vi "RangeCheck.vi"(8 "error in (no error)":errorcluster caption="エラー入力（エラーなし）", 10 "数値範囲チェック":T1={"デフォルト"=2.0, "最大値"=1.0, "最小値"=0.0}, 11 "数値文字列":string="0") -> (0 "error out":errorcluster caption="エラー出力", 2 "強制(x)":dbl, 3 "範囲内?(有効:TRUE,無効:FALSE)":bool)   [LabVIEW 2015]
uses:
  RangeCheck.ctl
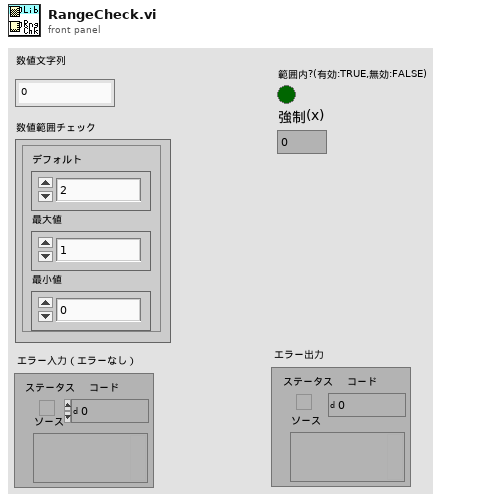
[diagram p1: front panel]
types:
  T1 = typedef "RangeCheck.ctl" = cluster{"デフォルト":dbl, "最大値":dbl, "最小値":dbl}
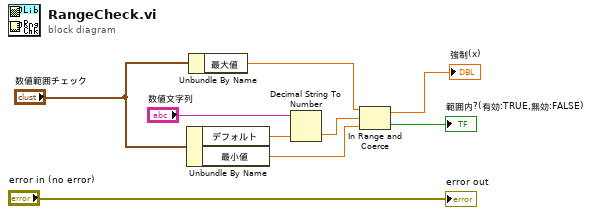
[diagram p0: block diagram]
diagram:
  n1 = Unbundle By Name("数値範囲チェック") -> ("デフォルト"=w9:dbl, "最小値"=w7:dbl)
  n2 = Unbundle By Name("数値範囲チェック") -> ("最大値"=w8:dbl)
  n3 = Decimal String To Number(string="数値文字列", default (0L)=w9) -> (number=w6:dbl)  [unwired: 1 in, 1 out]
  n4 = In Range and Coerce(upper limit=w8, x=w6, lower limit=w7) -> (coerced(x)=→"強制(x)":dbl, In Range?=→"範囲内?(有効:TRUE,無効:FALSE)":bool)
  "error out" <- "error in (no error)"
